vi "Polar Plot Property Pages.vi"(3 "Display State In":T1={"Plot Attributes"={"maximum"=2.0, "minimum"=0.0, "clip to min"=FALSE, "log"=FALSE, "grid color"=3381657, "plot color"=16711680, "fmt and prec"={"format"=enum."Decimal", "precision"=2}, "visible section"=4}, "Desired Font"=enum."Application Font", "User-Specified Font"={"Font Name:"="monaco", "Size"=9, "Strikeout?"=FALSE, "Italic?"=FALSE, "Underline?"=FALSE, "Outline?"=FALSE, "Shadow?"=FALSE, "Bold?"=FALSE}} {"Plot Attributes"."minimum" format="%0.2f"; "Plot Attributes"."maximum" format="%0.2f"}) -> (0 "OK?":bool, 1 "Display State Out":T1={"Plot Attributes"={"maximum"=2.0, "minimum"=0.0, "clip to min"=FALSE, "log"=FALSE, "grid color"=3381657, "plot color"=16711680, "fmt and prec"={"format"=enum."Decimal", "precision"=2}, "visible section"=4}, "Desired Font"=enum."Application Font", "User-Specified Font"={"Font Name:"="monaco", "Size"=9, "Strikeout?"=FALSE, "Italic?"=FALSE, "Underline?"=FALSE, "Outline?"=FALSE, "Shadow?"=FALSE, "Bold?"=FALSE}} {"Plot Attributes"."minimum" format="%0.2f"; "Plot Attributes"."maximum" format="%0.2f"})   [LabVIEW 2009, in "Polar Plot.xctl"]
doc: "Demonstration of an XControl.\n\nAAL 9/09"
uses:
  Polar Plot.xctl
panel:
  in  "Cancel":bool
  in  "OK":bool
  in  "Tab Control":enum32{"Appearance", "Scale", "Font"}(tab)
  in  "visible section":u16(ring)=4
  in  "Plot":u32(colorbox)=16711680
  in  "Grid":u32(colorbox)=46224
  in  "Precision":u8=2
  in  "Format:":u16(ring) items=["Decimal", "Scientific", "Engineering", "Binary", "Octal", "Hex"]
  in  "log":bool
  in  "clip":bool
  in  "Maximum":dbl=2.0
  in  "Minimum":dbl
  in  "UserFont":T2={"Font Name"="Arial", "Size"=9.0, "Strikeout"=FALSE, "Italic"=FALSE, "Underline"=FALSE, "Outline"=FALSE, "Bold"=FALSE, "Shadow"=FALSE}
  in  "Style":u16(ring)=1 items=["User-specified Font", "Application Font", "System Font", "Dialog Font"]
  # "Colors"
  # "Visible Section"
  # "Range"
  # "Format & Precision"
  # "User Specifed Font"
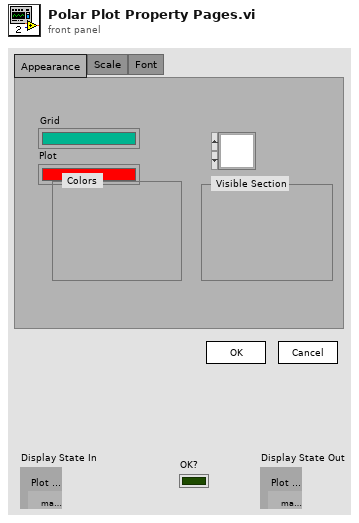
[diagram p1: front panel]
types:
  T1 = cluster{"Plot Attributes":cluster{"maximum":dbl, "minimum":dbl, "clip to min":bool, "log":bool, "grid color":u32, "plot color":u32, "fmt and prec":cluster{"format":enum8{"Decimal", "Scientific", "Engineering", "Binary", "Octal", "Hex"}, "precision":u8}, "visible section":u16}, "Desired Font":enum16{"User-specified Font", "Application Font", "System Font", "Dialog Font"}, "User-Specified Font":cluster{"Font Name:":string, "Size":i16, "Strikeout?":bool, "Italic?":bool, "Underline?":bool, "Outline?":bool, "Shadow?":bool, "Bold?":bool}}
  T2 = cluster{"Font Name":string, "Size":dbl, "Strikeout":bool, "Italic":bool, "Underline":bool, "Outline":bool, "Bold":bool, "Shadow":bool}
  T3 = enum8{"Decimal", "Scientific", "Engineering", "Binary", "Octal", "Hex"}
  T4 = enum16{"User-specified Font", "Application Font", "System Font", "Dialog Font"}
  T5 = cluster{"Font Name:":string, "Size":i16, "Strikeout?":bool, "Italic?":bool, "Underline?":bool, "Outline?":bool, "Shadow?":bool, "Bold?":bool}
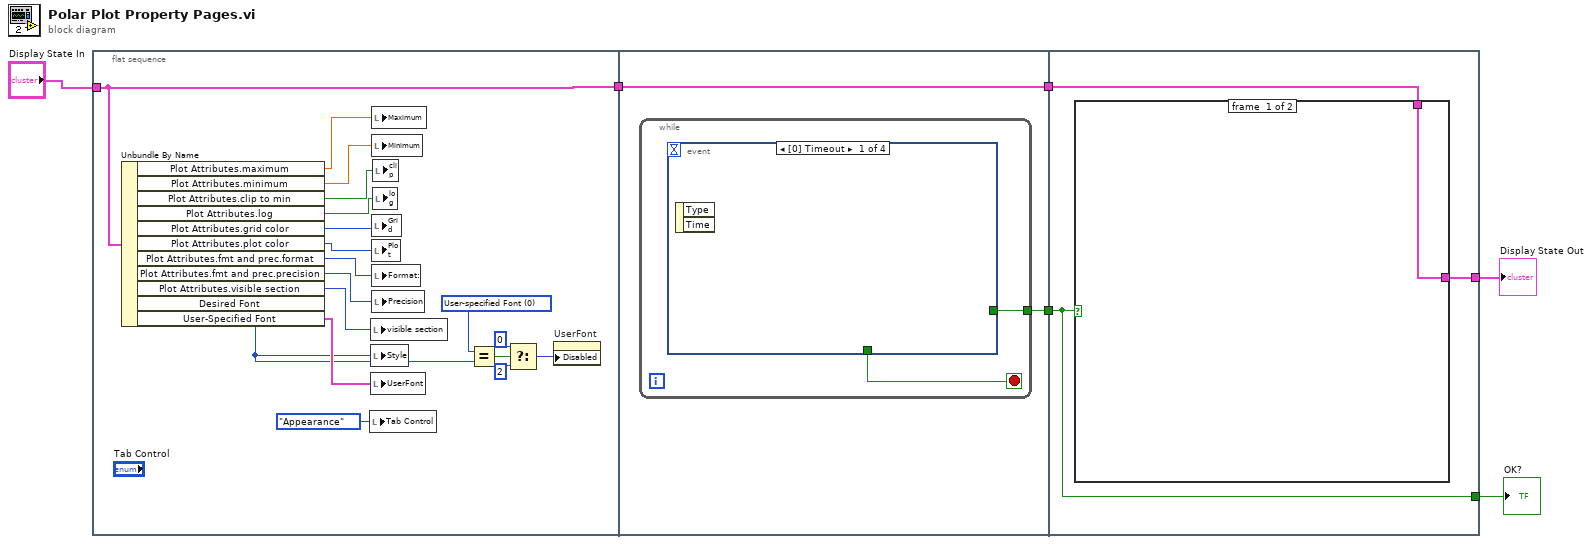
[diagram p0: block diagram]
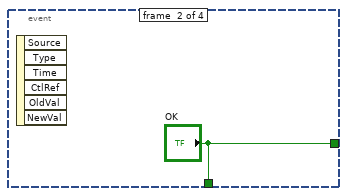
[diagram p2: hidden frame]
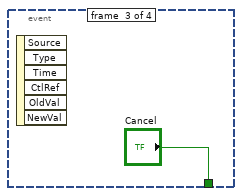
[diagram p3: hidden frame]
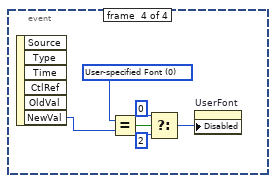
[diagram p4: hidden frame]
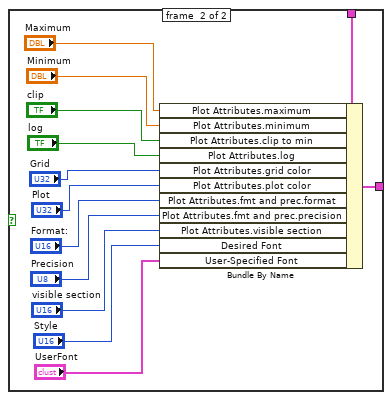
[diagram p5: hidden frame]
diagram:
  n1 = flat-sequence {
    tunnel: "Display State In" -> [w8]
    tunnel: [w8] -> w3
    tunnel: [w26] -> w5
    tunnel: [w25] -> w4
    tunnel: w3 -> [w25]
    tunnel: w5 -> [w37]
    tunnel: w4 -> [w39]
    tunnel: [w38] -> w2
    tunnel: [w37] -> w1
    frame #0 {
      w12 = u16 0 items=["User-specified Font", "Application Font", "System Font", "Dialog Font"] ("Style")
      n2 = Unbundle By Name(w8) -> ("Plot Attributes.maximum"=w24:dbl, "Plot Attributes.minimum"=w23:dbl, "Plot Attributes.clip to min"=w22:bool, "Plot Attributes.log"=w21:bool, "Plot Attributes.grid color"=w20:u32, "Plot Attributes.plot color"=w19:u32, "Plot Attributes.fmt and prec.format"=w18:T3, "Plot Attributes.fmt and prec.precision"=w17:u8, "Plot Attributes.visible section"=w16:u16, "Desired Font"=w13:T4, "User-Specified Font"=w15:T5)
      n3 = local write "Tab Control"(enum32{"Appearance", "Scale", "Font"}."Appearance" ("Tab Control")) -> ()
      n4 = local write "visible section"(w16) -> ()
      n5 = local write "Style"(w13) -> ()
      n6 = local write "UserFont"(w15) -> ()
      n7 = local write "Maximum"(w24) -> ()
      n8 = local write "Minimum"(w23) -> ()
      n9 = local write "Grid"(w20) -> ()
      n10 = local write "Plot"(w19) -> ()
      n11 = local write "Format:"(w18) -> ()
      n12 = local write "Precision"(w17) -> ()
      n13 = local write "clip"(w22) -> ()
      n14 = local write "log"(w21) -> ()
      n15 = Equal?(x=w12, y=w13) -> (x = y?=w14:bool)
      n16 = Select(t=0, s=w14, f=2) -> (s? t:f=w9:i32)
      n17 = property on="UserFont" class="Clust (strict)"("Disabled"=w9) -> ()  [unwired: 2 in, 2 out]
    }
    frame #1 {
      n18 = while {
        tunnel: [w27] -> w26
        stop <- w28 stop-if-true
        n19 = event shown="[0] Timeout" {
          selector: _ -> [_ _ _ _]
          dyn-events: _ -> [_ _ _ _]
          timeout: _ -> [_ _ _ _]
          tunnel: [_ "OK" "Cancel" _] -> w28
          tunnel: [_ "OK" _ _] -> w27
          event #0 {
            n20 = event-data() -> ()  [unwired: 1 in, 2 out]
          }
          event #1 {
            n21 = event-data() -> ()  [unwired: 1 in, 6 out]
          }
          event #2 {
            n22 = event-data() -> ()  [unwired: 1 in, 6 out]
          }
          event #3 {
            w33 = u16 0 items=["User-specified Font", "Application Font", "System Font", "Dialog Font"] ("Style")
            n23 = event-data() -> ("NewVal"=w31:u16)  [unwired: 1 in, 5 out]
            n24 = Equal?(x=w33, y=w31) -> (x = y?=w32:bool)
            n25 = Select(t=0, s=w32, f=2) -> (s? t:f=w36:i32)
            n26 = property on="UserFont" class="Clust (strict)"("Disabled"=w36) -> ()  [unwired: 2 in, 2 out]
          }
        }
      }
    }
    frame #2 {
      n27 = case shown="True" w37 {
        tunnel: w39 -> [w40 w53]
        tunnel: [w40 w52] -> w38
        frame #0 {
        }
        frame #1 {
          n28 = Bundle By Name(cluster=w53, "Plot Attributes.maximum"="Maximum", "Plot Attributes.minimum"="Minimum", "Plot Attributes.clip to min"="clip", "Plot Attributes.log"="log", "Plot Attributes.grid color"="Grid", "Plot Attributes.plot color"="Plot", "Plot Attributes.fmt and prec.format"="Format:", "Plot Attributes.fmt and prec.precision"="Precision", "Plot Attributes.visible section"="visible section", "Desired Font"="Style", "User-Specified Font"="UserFont") -> (w52:T1)
        }
      }
    }
  }
  "Display State Out" <- w2
  "OK?" <- w1
